vi "Read UI Constants.vi"(8 "error in":errorcluster, 11 "CFG File Refnum in":T2) -> (0 "error out":errorcluster, 2 "MHL Configuration":T1, 3 "CFG File Refnum out":T2)   [LabVIEW 2014]
uses:
  <vilib>/Utility/config.llb/Config Data RefNum.ctl
  controls/MHL Configuration.ctl
  Boiler System Globals.vi
  <vilib>/Utility/config.llb/Read Key (Double).vi
  <vilib>/Utility/config.llb/NI_LVConfig.lvlib
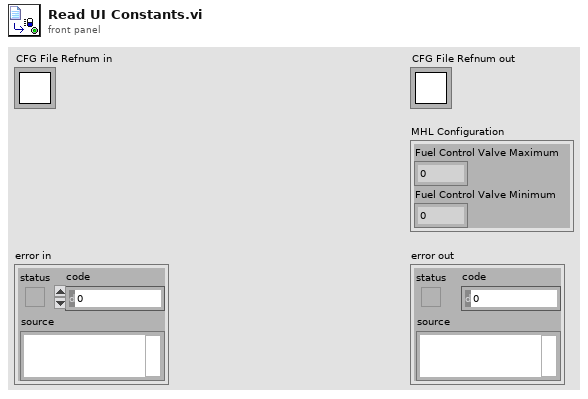
[diagram p1: front panel]
types:
  T1 = typedef "MHL Configuration.ctl" = cluster{"Fuel Control Valve Maximum":dbl, "Fuel Control Valve Minimum":dbl}
  T2 = typedef "NI_LVConfig.lvlib/Config Data RefNum.ctl" = refnum<k1>
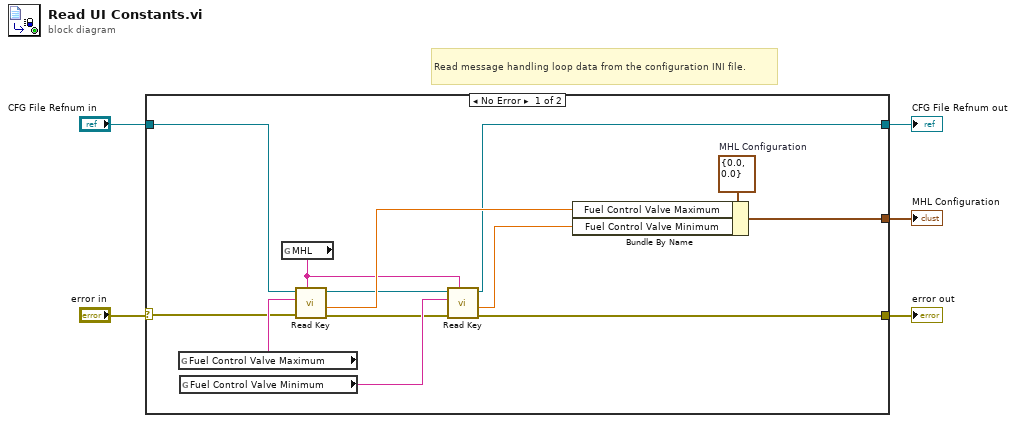
[diagram p0: block diagram]
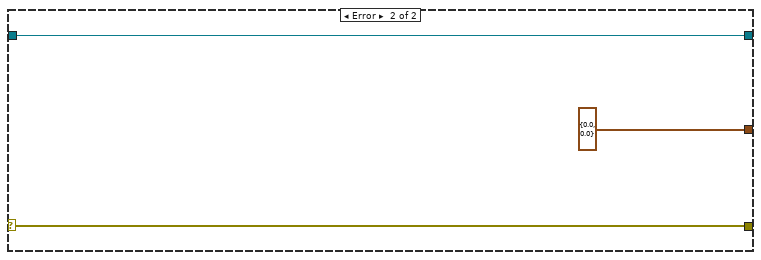
[diagram p2: hidden frame]
diagram:
  # "Read message handling loop data from the configuration INI file."
  n1 = case shown="No Error" "error in" {
    selector: "error in" -> [w16 w20]
    tunnel: "CFG File Refnum in" -> [w17 w21]
    tunnel: [w10 w20] -> w4
    tunnel: [w7 w21] -> w3
    tunnel: [w13 T1 {"Fuel Control Valve Maximum"=0.0, "Fuel Control Valve Minimum"=0.0} ("MHL Configuration Data")] -> w1
    frame No Error {
      w15 = T1 {"Fuel Control Valve Maximum"=0.0, "Fuel Control Valve Minimum"=0.0}  # MHL Configuration
      n2 = global read "Boiler System Globals.vi" "Fuel Control Valve Maximum"() -> (w18:string)
      n3 = global read "Boiler System Globals.vi" "Fuel Control Valve Minimum"() -> (w12:string)
      n4 = global read "Boiler System Globals.vi" "MHL"() -> (w9:string)
      n5 = call-poly <vilib>:"Read Key.vi"("section"=w9, "error in (no error)"=w16, "key"=w18, "refnum"=w17) -> ("error out"=w11:errorcluster, "value"=w14:dbl, "refnum out"=w8:T2)  [unwired: 4 in, 1 out]
      n6 = call-poly <vilib>:"Read Key.vi"("section"=w9, "error in (no error)"=w11, "key"=w12, "refnum"=w8) -> ("error out"=w10:errorcluster, "value"=w6:dbl, "refnum out"=w7:T2)  [unwired: 4 in, 1 out]
      n7 = Bundle By Name(cluster=w15, "Fuel Control Valve Maximum"=w14, "Fuel Control Valve Minimum"=w6) -> (w13:T1)
    }
    frame Error {
    }
  }
  "error out" <- w4
  "CFG File Refnum out" <- w3
  "MHL Configuration" <- w1
